vi "getRegisters.vi"(0 "AddressSpace in":refnum<class "AddressSpace.lvclass">) -> (4 "AddressSpace out":refnum<class "AddressSpace.lvclass">, 6 "Parameters":T1={"ReversePolarity"="ReversePolarity", "dTPerSec"="dTPerSec", "RevPerPulse"="RevPerPulse", "dT"="dT"})   [LabVIEW 2015, in "QuadEnc.lvlib" / "AddressSpace.lvclass"]
uses:
  AddressSpace.lvclass
  Parameters.ctl
  AddressSpace.lvclass/AddressSpace.ctl
  QuadEnc.lvlib
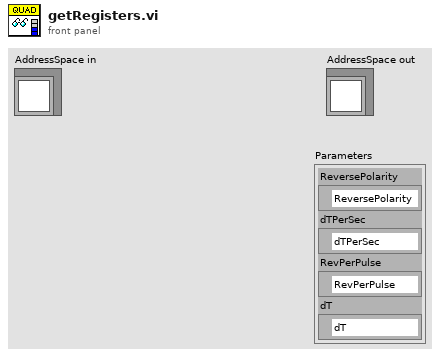
[diagram p1: front panel]
types:
  T1 = typedef "QuadEnc.lvlib/Parameters.ctl" = cluster{"ReversePolarity":refnum<k21>, "dTPerSec":refnum<k21>, "RevPerPulse":refnum<k21>, "dT":refnum<k21>}
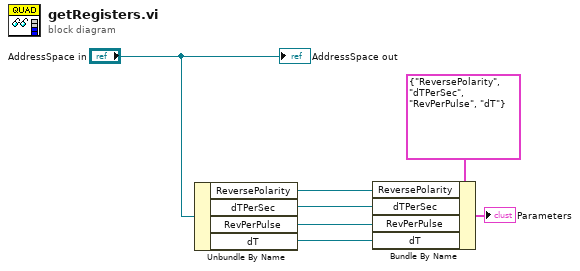
[diagram p0: block diagram]
diagram:
  n1 = Unbundle By Name("AddressSpace in") -> ("ReversePolarity"=w5:refnum<k21>, "dTPerSec"=w4:refnum<k21>, "RevPerPulse"=w3:refnum<k21>, "dT"=w2:refnum<k21>)
  n2 = Bundle By Name(cluster=T1 {"ReversePolarity"="ReversePolarity", "dTPerSec"="dTPerSec", "RevPerPulse"="RevPerPulse", "dT"="dT"} ("Parameters"), "ReversePolarity"=w5, "dTPerSec"=w4, "RevPerPulse"=w3, "dT"=w2) -> (→"Parameters":T1)
  "AddressSpace out" <- "AddressSpace in"
